vi "Simulation.Waveform.vi"(0 "Temperatur 1 [°C]":dbl, 1 "Temperatur 2 [°C]":dbl, 2 "Temperatur 3 [°C]":dbl, 3 "Temperatur 4 [°C]":dbl, 4 "Temperatur 5 [°C]":dbl, 5 "Temperatur 6 [°C]":dbl, 7 "Temperatur 7 [°C]":dbl, 9 "Zeit":timestamp) -> (17 "Waveform Chart":waveform(dbl)[](graph))   [LabVIEW 2016, in "Simulation.lvclass"]
uses:
  Simulation.lvclass
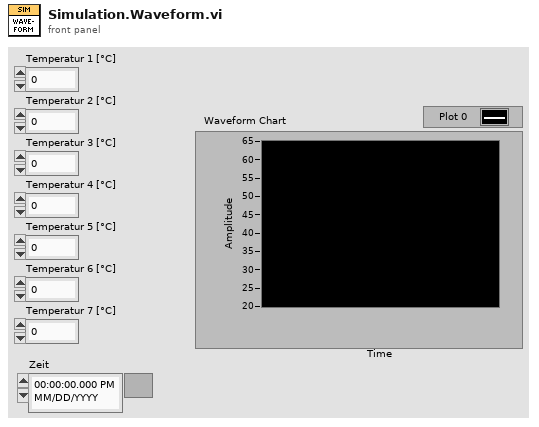
[diagram p1: front panel]
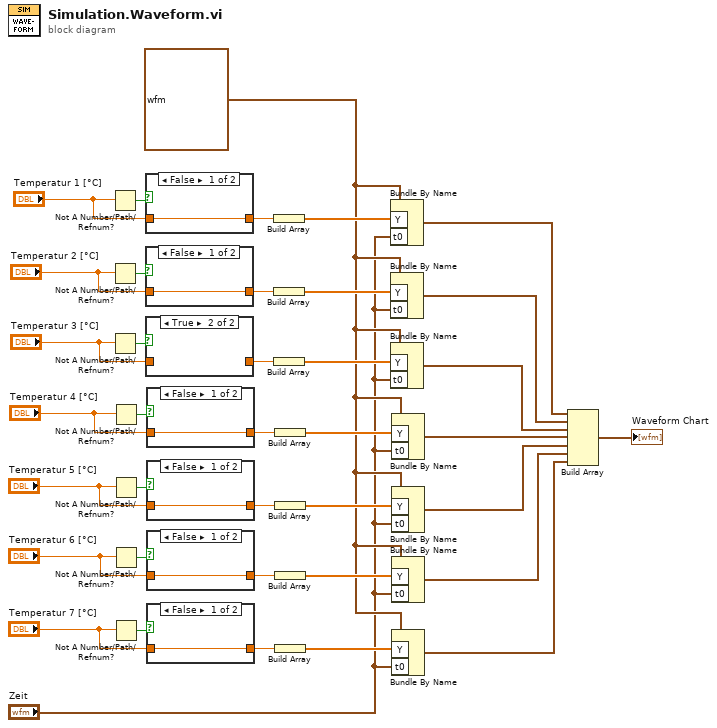
[diagram p0: block diagram]
diagram:
  w10 = waveform(dbl) {"t0"=timestamp(0 s since 1904-01-01), "dt"=1.0, "Y"=[]} ("waveform")
  n1 = Not A Number/Path/Refnum?(number/path/refnum="Temperatur 1 [°C]") -> (NaN/Path/Refnum?=w16:bool)
  n2 = Not A Number/Path/Refnum?(number/path/refnum="Temperatur 2 [°C]") -> (NaN/Path/Refnum?=w19:bool)
  n3 = Not A Number/Path/Refnum?(number/path/refnum="Temperatur 3 [°C]") -> (NaN/Path/Refnum?=w22:bool)
  n4 = Not A Number/Path/Refnum?(number/path/refnum="Temperatur 4 [°C]") -> (NaN/Path/Refnum?=w28:bool)
  n5 = Not A Number/Path/Refnum?(number/path/refnum="Temperatur 5 [°C]") -> (NaN/Path/Refnum?=w31:bool)
  n6 = Not A Number/Path/Refnum?(number/path/refnum="Temperatur 6 [°C]") -> (NaN/Path/Refnum?=w34:bool)
  n7 = Not A Number/Path/Refnum?(number/path/refnum="Temperatur 7 [°C]") -> (NaN/Path/Refnum?=w38:bool)
  n8 = case shown="False" w16 {
    tunnel: "Temperatur 1 [°C]" -> [w39 _]
    tunnel: [w39 _] -> w15
    frame False {
    }
    frame True {
    }
  }
  n9 = case shown="False" w19 {
    tunnel: "Temperatur 2 [°C]" -> [w40 _]
    tunnel: [w40 _] -> w18
    frame False {
    }
    frame True {
    }
  }
  n10 = case shown="True" w22 {
    tunnel: "Temperatur 3 [°C]" -> [w41 _]
    tunnel: [w41 _] -> w21
    frame False {
    }
    frame True {
    }
  }
  n11 = case shown="False" w28 {
    tunnel: "Temperatur 4 [°C]" -> [w42 _]
    tunnel: [w42 _] -> w27
    frame False {
    }
    frame True {
    }
  }
  n12 = case shown="False" w31 {
    tunnel: "Temperatur 5 [°C]" -> [w43 _]
    tunnel: [w43 _] -> w30
    frame False {
    }
    frame True {
    }
  }
  n13 = case shown="False" w34 {
    tunnel: "Temperatur 6 [°C]" -> [w44 _]
    tunnel: [w44 _] -> w33
    frame False {
    }
    frame True {
    }
  }
  n14 = case shown="False" w38 {
    tunnel: "Temperatur 7 [°C]" -> [w45 _]
    tunnel: [w45 _] -> w36
    frame False {
    }
    frame True {
    }
  }
  n15 = Build Array(w15) -> (w14:dbl[])
  n16 = Build Array(w18) -> (w17:dbl[])
  n17 = Build Array(w21) -> (w20:dbl[])
  n18 = Build Array(w27) -> (w26:dbl[])
  n19 = Build Array(w30) -> (w29:dbl[])
  n20 = Build Array(w33) -> (w32:dbl[])
  n21 = Build Array(w36) -> (w35:dbl[])
  n22 = Bundle By Name(cluster=w10, "Y"=w14, "t0"="Zeit") -> (w5:waveform(dbl))
  n23 = Bundle By Name(cluster=w10, "Y"=w17, "t0"="Zeit") -> (w6:waveform(dbl))
  n24 = Bundle By Name(cluster=w10, "Y"=w20, "t0"="Zeit") -> (w7:waveform(dbl))
  n25 = Bundle By Name(cluster=w10, "Y"=w26, "t0"="Zeit") -> (w8:waveform(dbl))
  n26 = Bundle By Name(cluster=w10, "Y"=w29, "t0"="Zeit") -> (w4:waveform(dbl))
  n27 = Bundle By Name(cluster=w10, "Y"=w32, "t0"="Zeit") -> (w3:waveform(dbl))
  n28 = Bundle By Name(cluster=w10, "Y"=w35, "t0"="Zeit") -> (w2:waveform(dbl))
  n29 = Build Array(w5, w6, w7, w8, w4, w3, w2) -> (→"Waveform Chart":waveform(dbl)[])
